vi "First Step.vi"(8 "error in (no error)":errorcluster, 11 "Translation Stage.lvclass in":refnum<class "Translation Stage.lvclass">) -> (0 "error out":errorcluster, 2 "Current Position":dbl, 3 "Translation Stage.lvclass out":refnum<class "Translation Stage.lvclass">)   [LabVIEW 2017, in "Translation Stage.lvclass"]
doc: "Goto step #0 - the first step. If desired, the scanner may do this in a different way than usual (i.e. by preparing to move a long distance, or reset to home position.)"
uses:
  Translation Stage.lvclass
  Translation Stage.lvclass/Translation Stage.ctl
  Global/GPIB Numbers.vi
  Scanner/Scanner.lvclass
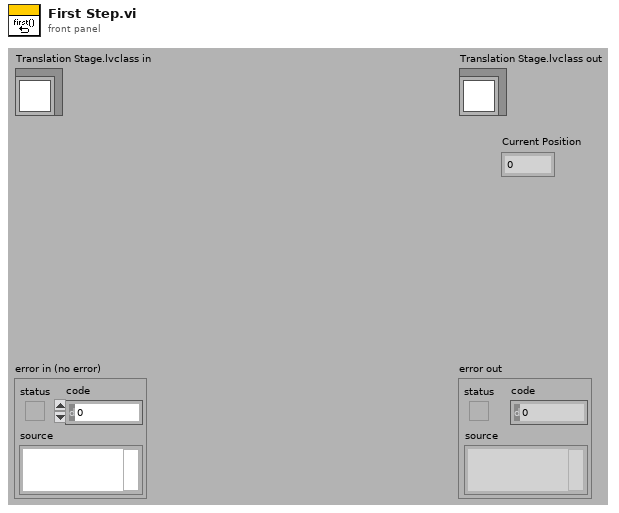
[diagram p1: front panel]
types:
  T1 = typedef "GPIB Type Def.ctl" = cluster{"Name":string, "bus":dbl, "GPIB":dbl, "GPIB as string":string, "byte":i32, "VISA Resource Name":refnum<visa-resource-name>}
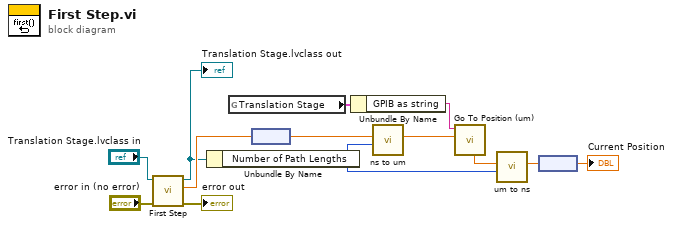
[diagram p0: block diagram]
diagram:
  n1 = call-parent "First Step.vi"("error in (no error)"="error in (no error)", "Scanner.lvclass in"="Translation Stage.lvclass in") -> ("error out"=→"error out":errorcluster, "Current Position"=w9:dbl, "Scanner.lvclass out"=w4:refnum<class "Translation Stage.lvclass">)  [unwired: 7 out]
  "Translation Stage.lvclass out" <- w4
  n2 = Unbundle By Name(w4) -> ("Number of Path Lengths"=w3:i32)
  n3 = global read "GPIB Numbers.vi" "Translation Stage"() -> (w2:T1)
  n4 = node(w9) -> (w10:dbl[unit])
  n5 = Unbundle By Name(w2) -> ("GPIB as string"=w1:string)
  n6 = call "ns to um.vi"("number of path lengths (default: 2)"=w3, "position (ns)"=w10) -> ("position (microns)"=w8:dbl[unit])  [unwired: 9 out]
  n7 = call "Go To Position (um).vi"("Position (um)"=w8, "GPIB # (in): def. 6"=w1) -> ("combined position (um)"=w6:ext[unit])  [unwired: 1 in, 8 out]
  n8 = call "um to ns.vi"("# of path lengths (def.: 2)"=w3, "position (microns)"=w6) -> ("position (ns)"=w5:dbl[unit])  [unwired: 9 out]
  n9 = node(w5) -> (→"Current Position":dbl)
